vi "Robot Status Checker.vi"() -> ()   [LabVIEW 2015]
uses:
  <vilib>/httpClient/LabVIEWHTTPClient.lvlib
panel:
  in  "?":bool
  in  "Turn On Checker":bool
  out "?":bool
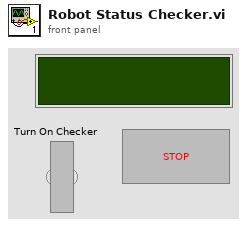
[diagram p1: front panel]
types:
  T1 = typedef "LabVIEWHTTPClient.lvlib/ClientHandle.ctl" = refnum<k1>
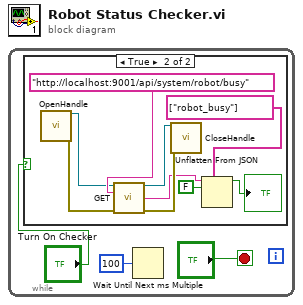
[diagram p0: block diagram]
diagram:
  n1 = while {
    stop <- "?" stop-if-true
    n2 = case shown="True" "Turn On Checker" {
      frame False {
      }
      frame True {
        n3 = call <vilib>:"OpenHandle.vi"() -> ("client handle out"=w11:T1, "error out"=w10:errorcluster)  [unwired: 14 in]
        n4 = call <vilib>:"GET.vi"("client handle"=w11, "url"="http://localhost:9001/api/system/robot/busy", "error in (no error)"=w10) -> ("client handle out"=w9:T1, "body"=w4:string, "error out"=w8:errorcluster)  [unwired: 9 in, 1 out]
        n5 = call <vilib>:"CloseHandle.vi"("client handle"=w9, "error in (no error)"=w8) -> ()  [unwired: 13 in, 1 out]
        n6 = Unflatten From JSON(path=string[] ["robot_busy"], JSON string=w4, type and defaults=FALSE) -> (value=→"?":bool)  [unwired: 4 in, 1 out]
      }
    }
    n7 = Wait Until Next ms Multiple(millisecond multiple=u32 100) -> ()  [unwired: 1 out]
  }
